vi "Write Dig Port.vi"() -> ()   [LabVIEW 2009]
doc: "I. Description:\nThis example demonstrates how to write values to a digital output port.\n\nII. Instructions for Running:\n1. Select the digital port on the DAQ device to be written.\n2. Select a value to write.\nNote: The Data to Write control is in hexadecimal.\n\nIII. Block Diagram Steps:\n1. Create a Digital Output channel. Use one channel for all lines. In this case, the port itself acts as an individual channel.\n2. Call the Start VI to start the task.\n3. Write digital port data in a loop until the user hits the stop button or an error occurs. This write VI writes a single sample of digital data on demand, so no timeout is necessary.\n4. Call the Clear Task VI to clear the Task.\n5. Use the popup dialog box to display an error or warning if any.\n\nIV. I/O Connections Overview:\nMake sure your signal output terminals match the Ports I/O Control. In this case wire the item to receive the signal to the first N digital lines on your DAQ Device."
uses:
  <vilib>/Utility/error.llb/DialogType.ctl
  <vilib>/DAQmx/create/channels.llb/DAQmx Create Channel (DO-Digital Output).vi
  <vilib>/DAQmx/write.llb/DAQmx Write (Digital U8 1Chan 1Samp).vi
panel:
  in  "Data to Write":u32=255 format="%x"
  in  "Port":tag="Dev1/port0"
  in  "stop":bool
  # "For instructions, select Help>>Show Context Help"
  # "Channel Parameters"
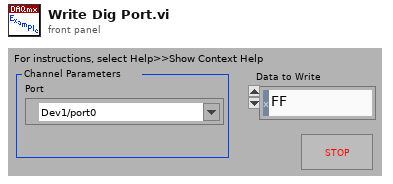
[diagram p1: front panel]
types:
  T1 = typedef "DialogType.ctl" = u16
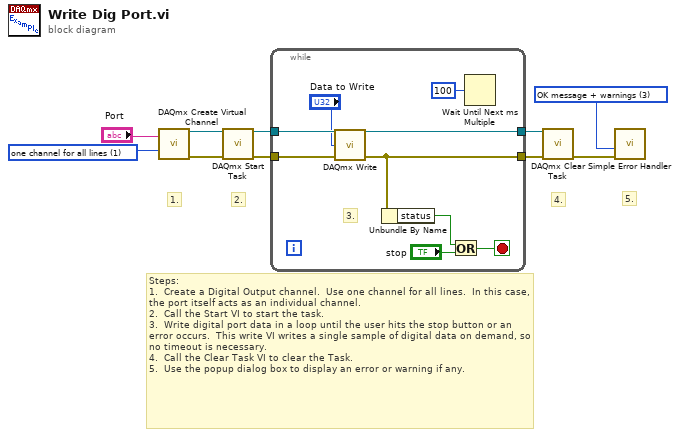
[diagram p0: block diagram]
diagram:
  w1 = 1 items=["one channel for each line", "one channel for all lines"] ("line grouping")
  w2 = T1 3 items=["no dialog", "OK message", "continue or stop message", "OK message + warnings", "continue/stop + warnings"] ("type of dialog (OK msg:1)")
  # "5."
  # "Steps: \n1.  Create a Digital Output channel.  Use one channel for all lines.  In this case, the port itself acts as an individual channel.\n2.  Call the Start VI to start the task.\n3.  Write digital port data in a loop until the user hits the stop button or an error occurs.  This write VI writes a single sample of digital data on demand, so no timeout is necessary.\n4.  Call the Clear Task VI to clear the Task.\n5.  Use the popup dialog box to display an error or warning if any."
  # "4."
  # "2."
  # "1."
  n1 = call-poly <vilib>:"DAQmx Create Virtual Channel.vi"("lines"="Port", "line grouping"=w1) -> ("task out"=w5:refnum<k21>, "error out"=w4:errorcluster)  [unwired: 12 in]
  n2 = call <vilib>:"DAQmx Start Task.vi"("task/channels in"=w5, "error in"=w4) -> ("task out"=w7:refnum<k21>, "error out"=w10:errorcluster)  [unwired: 12 in]
  n3 = while {
    tunnel: w10 -> [w19]
    tunnel: [w15] -> w9
    tunnel: w7 -> [w14]
    tunnel: [w13] -> w6
    stop <- w18 stop-if-true
    # "3."
    n4 = call-poly <vilib>:"DAQmx Write.vi"("task/channels in"=w14, "data"="Data to Write", "error in"=w19) -> ("task out"=w13:refnum<k21>, "error out"=w15:errorcluster)  [unwired: 10 in, 1 out]
    n5 = Unbundle By Name(w15) -> ("status"=w16:bool)
    n6 = Or(x=w16, y="stop") -> (x .or. y?=w18:bool)
    n7 = Wait Until Next ms Multiple(millisecond multiple=u32 100 ("milliseconds to wait")) -> ()  [unwired: 1 out]
  }
  n8 = call <vilib>:"DAQmx Clear Task.vi"("task in"=w6, "error in"=w9) -> ("error out"=w8:errorcluster)  [unwired: 13 in]
  n9 = call <vilib>:"Simple Error Handler.vi"("type of dialog (OK msg:1)"=w2, "error in (no error)"=w8) -> ()  [unwired: 3 in, 5 out]
